vi "All Data Save.vi"(6 "Cycel NO":u32, 7 "Ctl":T2(ring), 8 "error in (no error)":errorcluster caption="에러 입력(에러 없음)", 9 "Save.File Name":string, 11 "Q_data":T1) -> (0 "error out":errorcluster caption="에러 출력", 3 "Raw Data":dbl[][](array[numeric]))   [LabVIEW 2013]
uses:
  Ctrls/raw Q data.ctl
  <vilib>/Utility/xml.llb/Write to XML File(string).vi
  <vilib>/Utility/file.llb/Read From Spreadsheet File (DBL).vi
panel:
  out "dup path 3":path
  out "error out 2":errorcluster caption="에러 출력"
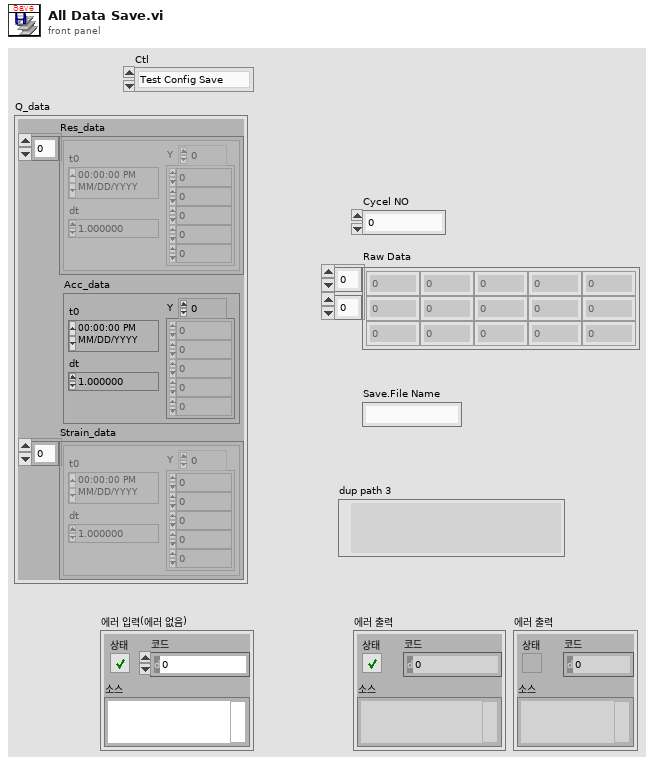
[diagram p1: front panel]
types:
  T1 = typedef "raw Q data.ctl" = cluster{"Res_data":waveform(dbl)[], "Acc_data":waveform(dbl), "Strain_data":waveform(dbl)[]}
  T2 = enum16{"Test Config Save", "Raw Data Save", "Raw Data Load"}
  T3 = cluster{"Test Information":cluster{"date":string, "custom":string, "oper":string, "package":string, "pkg side":string, "solder":string, "brd side":string, "paste":string, "reflow":string}, "Sensor Set":cluster{"Accelerometer":cluster{"Sensitivity(mV/g)":dbl}, "Strain Guage":cluster{"Ch.":dbl[], "Gage factor":dbl[], "Resistance":dbl[], "Poisson ratio":dbl[]}}, "Resistor Set":cluster{"Criterion Level":dbl, "Res. Set":cluster{"Res. Ch":dbl, "Res. Active":bool, "Res Initial":dbl}[]}, "Test Stop Condition":cluster{"Test cycle":u16, "Fail number in a cycle":u16, "Fail factor":cluster{"Duration":u16, "Fail No.":u16}}, "Acceleration Condition ":cluster{"Shock duration pecent [%]":u16}, "Save":cluster{"Save Path":path, "File Name":string}}
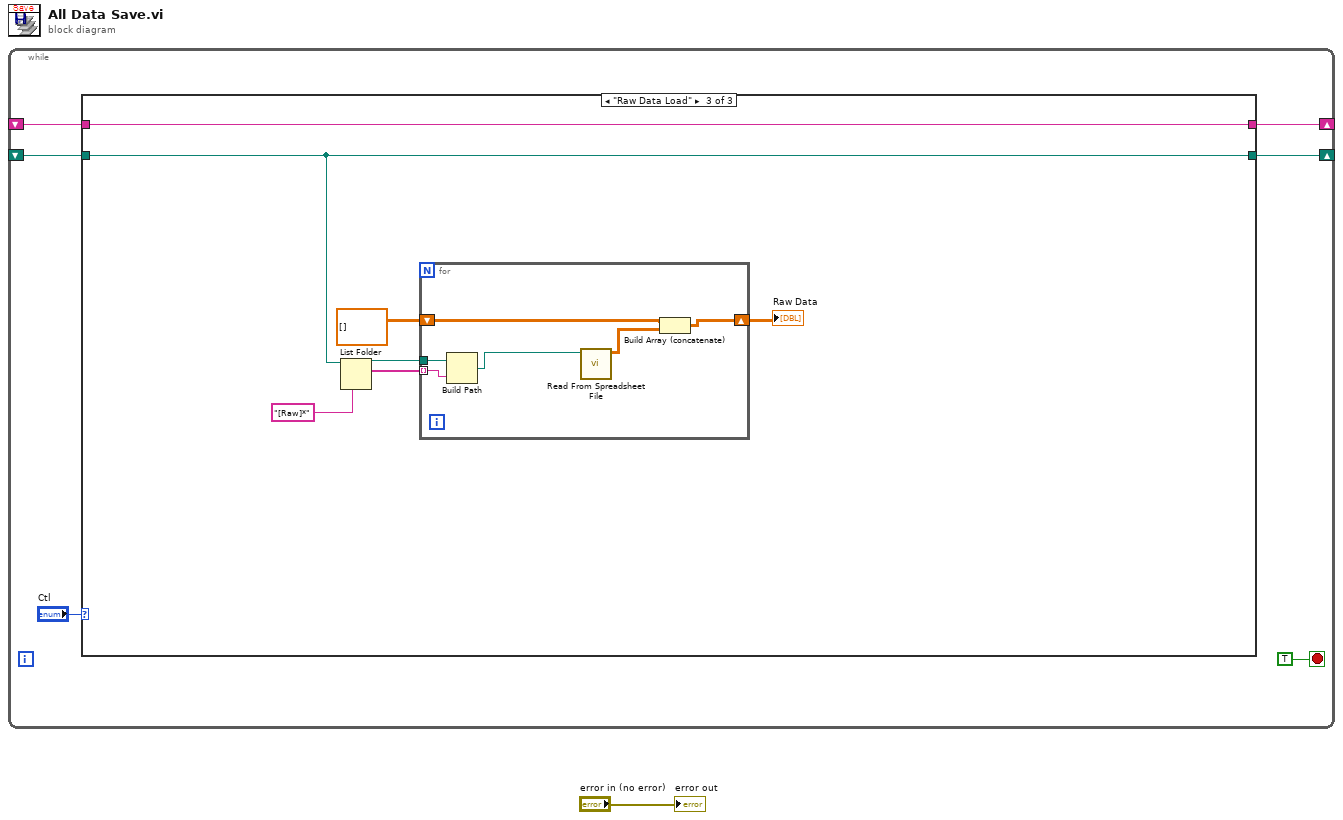
[diagram p0: block diagram]
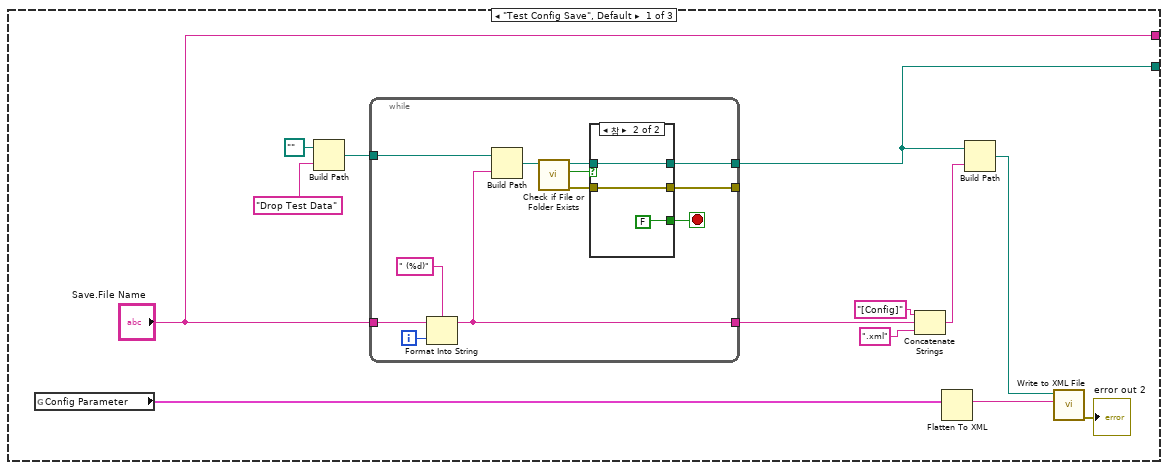
[diagram p2: hidden frame]
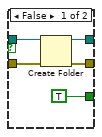
[diagram p3: hidden frame]
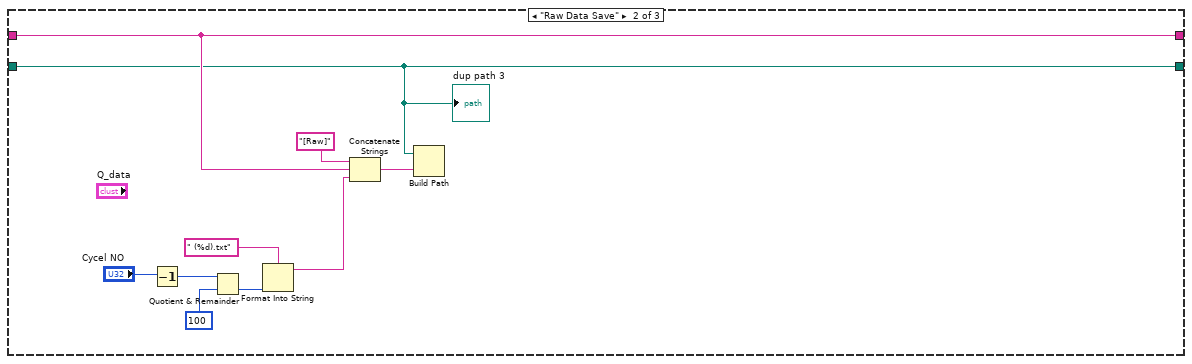
[diagram p4: hidden frame]
diagram:
  n1 = while {
    shift-right: [w6] -> _
    shift-left: _ -> [w4]
    shift-right: [w3] -> _
    shift-left: _ -> [w2]
    stop <- TRUE stop-if-true
    n2 = case shown="\"Raw Data Load\"" "Ctl" {
      tunnel: [w14 w41 w56] -> w6
      tunnel: w4 -> [_ w41 w56]
      tunnel: ["Save.File Name" w42 w57] -> w3
      tunnel: w2 -> [_ w42 w57]
      frame "Test Config Save", Default {
        n3 = global read "글로벌_Config Parameter.vi" "Config Parameter"() -> (w10:T3)
        n4 = Build Path(base path=path "" ("베이스 경로"), name or relative path="Drop Test Data" ("이름 또는 상대 경로")) -> (appended path=w13:path)
        n5 = while {
          tunnel: "Save.File Name" -> [w21]
          tunnel: [w26] -> _
          tunnel: [w24] -> w18
          tunnel: w13 -> [w31]
          tunnel: [w27] -> w14
          i -> [w32]
          stop <- w25 stop-if-true
          n6 = Format Into String(format string=" (%d)" ("포맷 문자열"), initial string=w21, w32) -> (resulting string=w24:string)  [unwired: 1 in, 1 out]
          n7 = Build Path(base path=w31, name or relative path=w24) -> (appended path=w30:path)
          n8 = call <vilib>:"Check if File or Folder Exists.vi"("path"=w30) -> ("error out"=w22:errorcluster, "file or folder exists?"=w28:bool, "dup path"=w29:path)  [unwired: 8 in]
          n9 = case shown="참" w28 {
            tunnel: w29 -> [w34 w40]
            tunnel: w22 -> [w33 w39]
            tunnel: [w37 w40] -> w27
            tunnel: [w36 w39] -> w26
            tunnel: [TRUE FALSE] -> w25
            frame False {
              n10 = Create Folder(path (use dialog)=w34, error in=w33) -> (created path=w37:path, error out=w36:errorcluster)  [unwired: 1 in, 1 out]
            }
            frame True {
            }
          }
        }
        n11 = Concatenate Strings("[Config]" ("문자열"), w18, ".xml" ("문자열")) -> (w19:string)
        n12 = Flatten To XML(anything=w10) -> (xml string=w11:string)
        n13 = Build Path(base path=w14, name or relative path=w19) -> (appended path=w15:path)
        n14 = call-poly <vilib>:"Write to XML File.vi"("XML Input"=w11, "XML File Path"=w15) -> ("error out"=→"error out 2":errorcluster)  [unwired: 7 in, 2 out]
      }
      frame "Raw Data Save" {
        n15 = Decrement(x="Cycel NO") -> (x-1=w47:u32)
        n16 = Quotient & Remainder(x=w47, y=u32 100) -> (floor(x/y)=w46:u32)  [unwired: 1 out]
        n17 = Format Into String(format string=" (%d).txt" ("포맷 문자열"), w46) -> (resulting string=w43:string)  [unwired: 2 in, 1 out]
        n18 = Concatenate Strings("[Raw]" ("문자열"), w42, w43) -> (w49:string)
        n19 = Build Path(base path=w41, name or relative path=w49) -> ()  [unwired: 1 out]
        "dup path 3" <- w41
      }
      frame "Raw Data Load" {
        n20 = List Folder(path=w56, pattern="[Raw]*" ("문자열")) -> (path out=w54:path, filenames=w53:string[])  [unwired: 2 in, 2 out]
        n21 = for {
          tunnel: w54 -> [w63]
          tunnel: w53 -> [w62] mode=indexing
          shift-right: [w59] -> w51
          shift-left: dbl[][] [] -> [w58]
          n22 = Build Path(base path=w63, name or relative path=w62) -> (appended path=w61:path)
          n23 = call-poly <vilib>:"Read From Spreadsheet File.vi"("file path (dialog if empty)"=w61) -> ("all rows"=w60:dbl[][])  [unwired: 6 in, 4 out]
          n24 = Build Array (concatenate)(w58, w60) -> (w59:dbl[][])
        }
        "Raw Data" <- w51
      }
    }
  }
  "error out" <- "error in (no error)"
